vi "Process XML Node.vi"(8 "error in (no error)":errorcluster, 11 "node in":refnum<k20>) -> (0 "error out":errorcluster, 1 "New Nodes":refnum<k20>[](array[refnum]), 2 "Data Item":refnum<class "Data Item.lvclass">, 3 "node out":refnum<k20>)   [LabVIEW 2026, in "VILab.lvlib"]
uses:
  VILab.lvlib
  <resource>/objmgr/DOMUserDefRef.rc
  Classes/Data Item/Data Item.lvclass
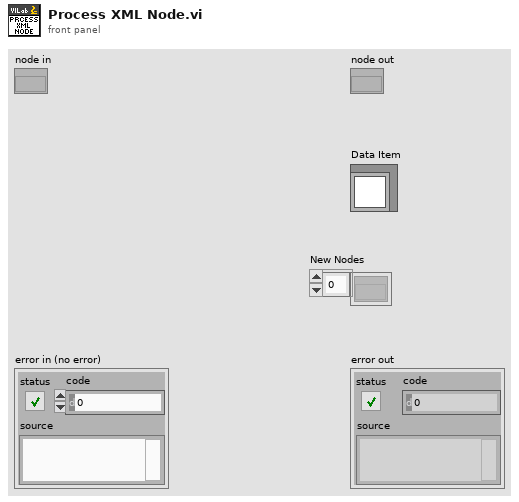
[diagram p1: front panel]
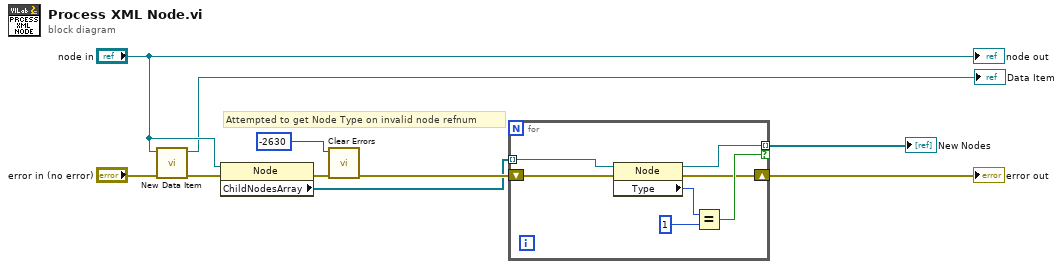
[diagram p0: block diagram]
diagram:
  # "Attempted to get Node Type on invalid node refnum"
  n1 = call "New Data Item.vi"("error in (no error)"="error in (no error)", "node in"="node in") -> ("error out"=w10:errorcluster, "Data Item"=→"Data Item":refnum<class "Data Item.lvclass">)  [unwired: 8 in]
  n2 = property class="Node"(reference="node in", error in=w10) -> (error out=w6:errorcluster, "ChildNodesArray"=w4:refnum<k20>[])  [unwired: 1 out]
  n3 = call <vilib>:"Clear Errors.vi"("error in (no error)"=w6, "specific error code to clear (0: all)"=-2630) -> ("error out"=w8:errorcluster)  [unwired: 4 in, 1 out]
  n4 = for {
    shift-right: [w11] -> w7
    shift-left: w8 -> [w17]
    tunnel: w4 -> [w16] mode=indexing
    tunnel: [w13] -> w1 mode=indexing if=w12
    n5 = property class="Node"(reference=w16, error in=w17) -> (reference out=w13:refnum<k20>, error out=w11:errorcluster, "Type"=w15:i32)
    n6 = Equal?(x=w15, y=1) -> (x = y?=w12:bool)
  }
  "error out" <- w7
  "New Nodes" <- w1
  "node out" <- "node in"
